vi "ge_FormatStringVals4GlblRing.vi"(0 "Values":u16[](array[numeric]), 1 "MeasType":T2, 2 "Hdr Name":T3, 4 "DefVal":u16=65535) -> (5 "String and Values":T1[](array[typedef]))   [LabVIEW 2012]
uses:
  Common/Controls/HeaderNames.ctl
  Custom Ctrls/ge_MeasType.ctl
  Custom Ctls Table/ge_StringVals.ctl
  Custom Ctls Table/ge_ColType.ctl
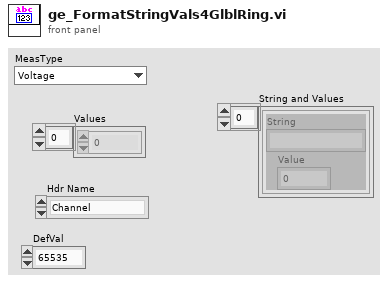
[diagram p1: front panel]
types:
  T1 = typedef "ge_StringVals.ctl" = cluster{"String":string, "Value":u16}
  T2 = typedef "ge_MeasType.ctl" = enum16{"Voltage", "Frequency", "Tachometer", "Dynamic", "Thermocouple", "RTD", "Strain", "Current", "Resistance"}
  T3 = typedef "HeaderNames.ctl" = enum16{"Channel", "Device", "Spacer", "Description", "MB", "Range", "Terminal", "Coupling", "Thresh (V)", "Pulse/Rev", "Slope", "Min EU", "Min RPM", "mV/EU", "Iex", "Temp Units", "Type", "CJC Src", "CJC Val", "Ro", "Wire Cfg", "Strain Mode", "Vex", "Bridge Type", "GF", "Gauge Res", "Poisson", "Lead Res", "Init Strain", "GAF", "Scale", "Offset", "Unit (EU)", "dB?", "dB Ref", "Cal Mag", "Cal Units", "Max Temp", "Min Temp", "Max Strain", "Min Strain"}
  T4 = typedef "ge_ColType.ctl" = enum16{"Volts", "Amps", "Ohms", "TermCfg", "WireCfg", "Coup", "Slope", "Iex", "CalUnits", "ThrmUnits", "ThrmType", "CJCSrc", "BrdgType", "Strn Mode", "RTDType"}
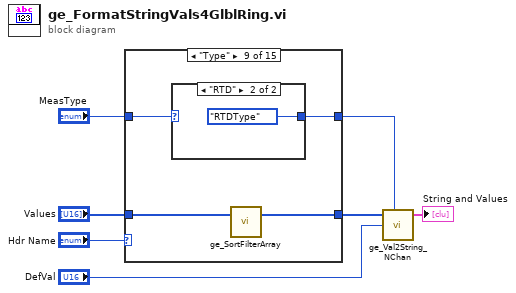
[diagram p0: block diagram]
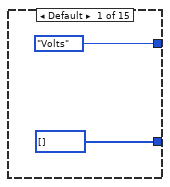
[diagram p2: hidden frame]
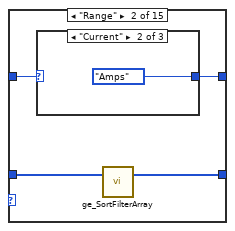
[diagram p3: hidden frame]
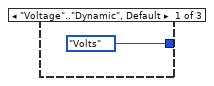
[diagram p4: hidden frame]
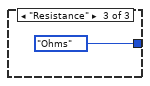
[diagram p5: hidden frame]
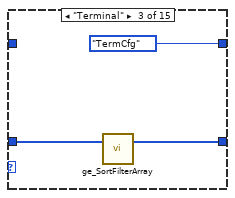
[diagram p6: hidden frame]
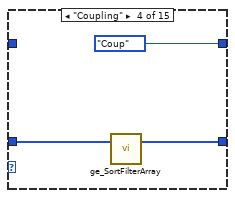
[diagram p7: hidden frame]
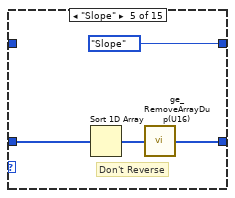
[diagram p8: hidden frame]
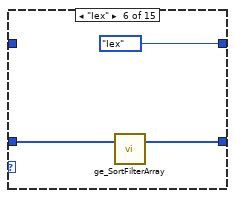
[diagram p9: hidden frame]
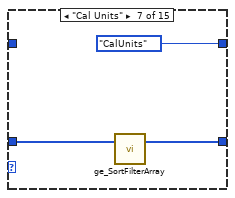
[diagram p10: hidden frame]
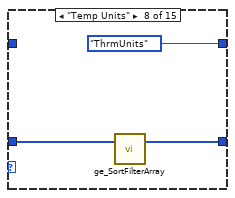
[diagram p11: hidden frame]
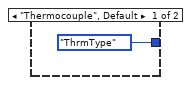
[diagram p12: hidden frame]
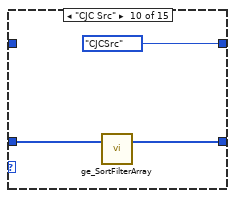
[diagram p13: hidden frame]
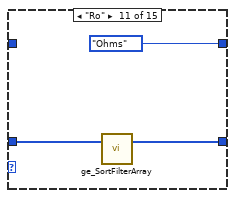
[diagram p14: hidden frame]
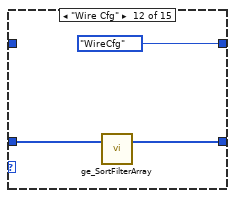
[diagram p15: hidden frame]
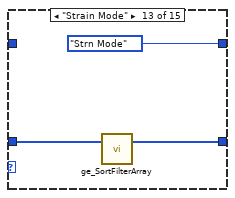
[diagram p16: hidden frame]
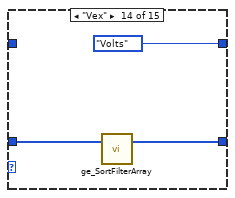
[diagram p17: hidden frame]
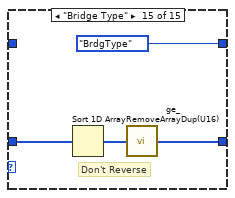
[diagram p18: hidden frame]
diagram:
  n1 = case shown="\"Type\"" "Hdr Name" {
    tunnel: "MeasType" -> [_ w13 _ _ _ _ _ _ w36 _ _ _ _ _ _]
    tunnel: "Values" -> [_ w12 w19 w22 w24 w28 w31 w34 w38 w44 w47 w50 w53 w56 w58]
    tunnel: [u16[] [] ("Array") w11 w18 w21 w23 w27 w30 w33 w37 w43 w46 w49 w52 w55 w57] -> w5
    tunnel: [ge_ColType."Volts" ("ColType") w10 ge_ColType."TermCfg" ("ColType") ge_ColType."Coup" ("ColType") ge_ColType."Slope" ("ColType") ge_ColType."Iex" ("ColType") ge_ColType."CalUnits" ("ColType") ge_ColType."ThrmUnits" ("ColType") w39 ge_ColType."CJCSrc" ("ColType") ge_ColType."Ohms" ("ColType") ge_ColType."WireCfg" ("ColType") ge_ColType."Strn Mode" ("ColType") ge_ColType."Volts" ("ColType") ge_ColType."BrdgType" ("ColType")] -> w7
    frame Default {
    }
    frame "Range" {
      n2 = case shown="\"Current\"" w13 {
        tunnel: [ge_ColType."Volts" ("ColType") ge_ColType."Amps" ("ColType") ge_ColType."Ohms" ("ColType")] -> w10
        frame "Voltage".."Dynamic", Default {
        }
        frame "Current" {
        }
        frame "Resistance" {
        }
      }
      n3 = call "ge_SortFilterArray.vi"("V Ranges"=w12) -> ("Array"=w11:u16[])  [unwired: 2 in]
    }
    frame "Terminal" {
      n4 = call "ge_SortFilterArray.vi"("V Ranges"=w19) -> ("Array"=w18:u16[])  [unwired: 2 in]
    }
    frame "Coupling" {
      n5 = call "ge_SortFilterArray.vi"("V Ranges"=w22) -> ("Array"=w21:u16[])  [unwired: 2 in]
    }
    frame "Slope" {
      # "Don't Reverse"
      n6 = Sort 1D Array(array=w24) -> (sorted array=w25:u16[])
      n7 = call "ge_RemoveArrayDup(U16).vi"("Input Array"=w25) -> ("Output Array"=w23:u16[])  [unwired: 4 in]
    }
    frame "Iex" {
      n8 = call "ge_SortFilterArray.vi"("V Ranges"=w28) -> ("Array"=w27:u16[])  [unwired: 2 in]
    }
    frame "Cal Units" {
      n9 = call "ge_SortFilterArray.vi"("V Ranges"=w31) -> ("Array"=w30:u16[])  [unwired: 2 in]
    }
    frame "Temp Units" {
      n10 = call "ge_SortFilterArray.vi"("V Ranges"=w34) -> ("Array"=w33:u16[])  [unwired: 2 in]
    }
    frame "Type" {
      n11 = case shown="\"RTD\"" w36 {
        tunnel: [ge_ColType."ThrmType" ("ColType") ge_ColType."RTDType" ("ColType")] -> w39
        frame "Thermocouple", Default {
        }
        frame "RTD" {
        }
      }
      n12 = call "ge_SortFilterArray.vi"("V Ranges"=w38) -> ("Array"=w37:u16[])  [unwired: 2 in]
    }
    frame "CJC Src" {
      n13 = call "ge_SortFilterArray.vi"("V Ranges"=w44) -> ("Array"=w43:u16[])  [unwired: 2 in]
    }
    frame "Ro" {
      n14 = call "ge_SortFilterArray.vi"("V Ranges"=w47) -> ("Array"=w46:u16[])  [unwired: 2 in]
    }
    frame "Wire Cfg" {
      n15 = call "ge_SortFilterArray.vi"("V Ranges"=w50) -> ("Array"=w49:u16[])  [unwired: 2 in]
    }
    frame "Strain Mode" {
      n16 = call "ge_SortFilterArray.vi"("V Ranges"=w53) -> ("Array"=w52:u16[])  [unwired: 2 in]
    }
    frame "Vex" {
      n17 = call "ge_SortFilterArray.vi"("V Ranges"=w56) -> ("Array"=w55:u16[])  [unwired: 2 in]
    }
    frame "Bridge Type" {
      # "Don't Reverse"
      n18 = Sort 1D Array(array=w58) -> (sorted array=w59:u16[])
      n19 = call "ge_RemoveArrayDup(U16).vi"("Input Array"=w59) -> ("Output Array"=w57:u16[])  [unwired: 4 in]
    }
  }
  n20 = call "ge_Val2String_NChan.vi"("Values"=w5, "ColType"=w7, "DefVal"="DefVal") -> ("String and Values"=→"String and Values":cluster{"String":string, "Value":u16}[])  [unwired: 4 in]
